vi "get_nxsp.vi"(5 "lc_num":string, 6 "yw":string, 7 "id":string, 9 "Cur_state":string, 11 "fqren":string) -> (1 "nx_state":dbl, 2 "sp_name":string, 3 "sp_gonghao":string)   [LabVIEW 2017, in "Lib_code.lvlib"]
uses:
  Lib_code.lvlib
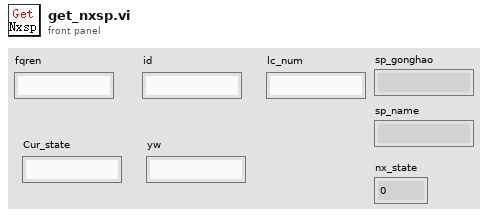
[diagram p1: front panel]
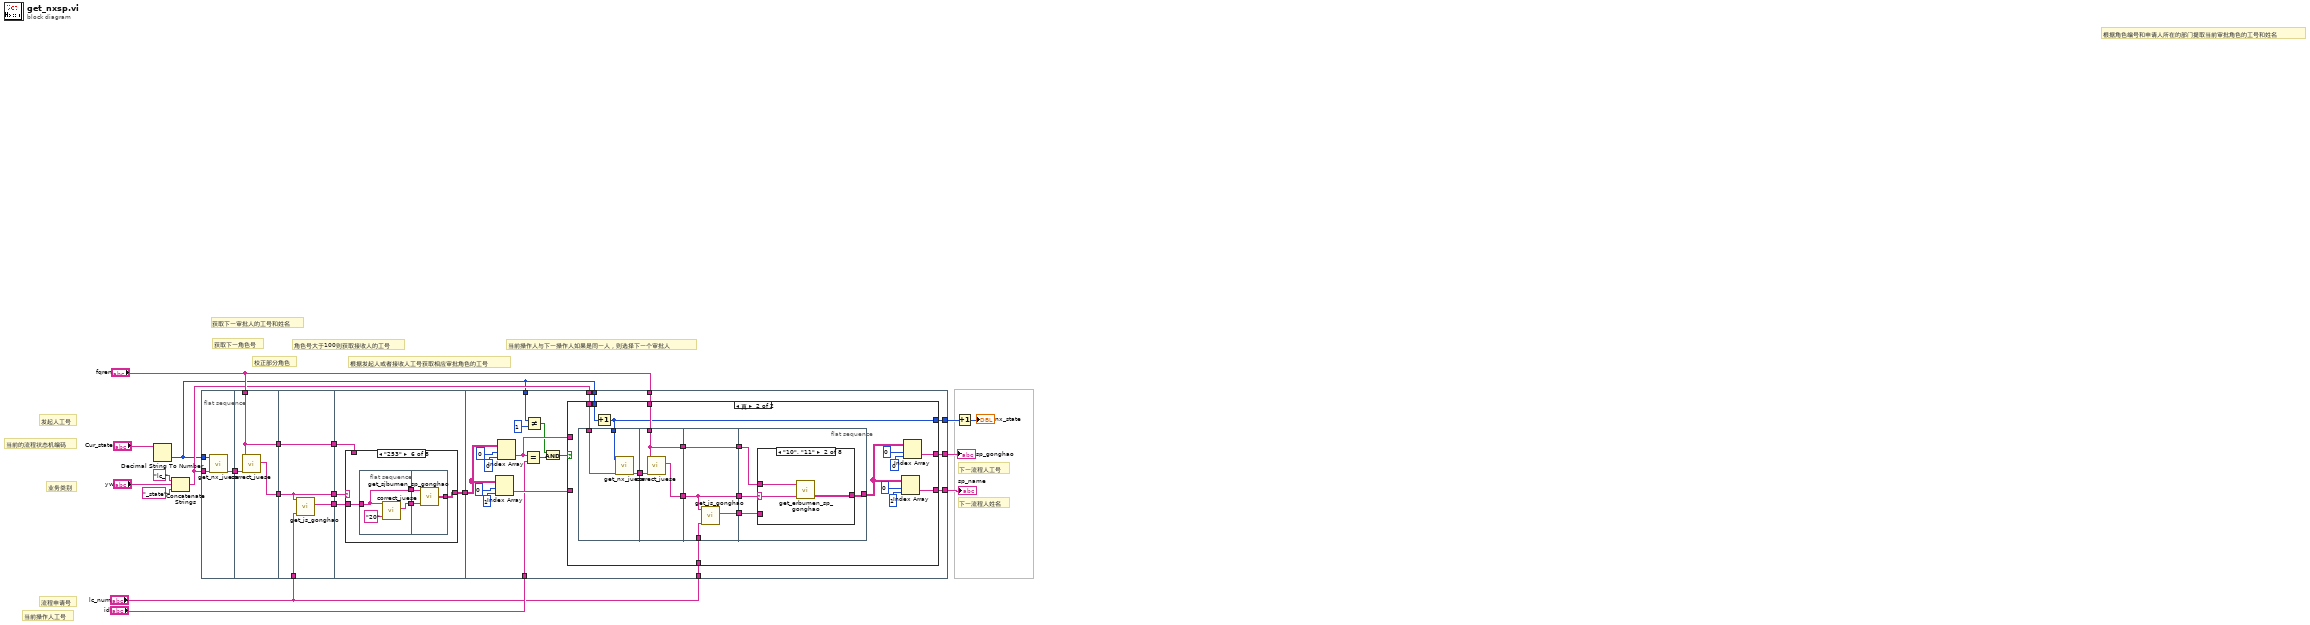
[diagram p0: block diagram]
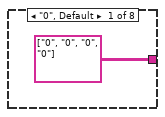
[diagram p2: hidden frame]
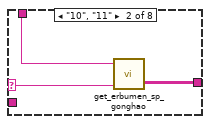
[diagram p3: hidden frame]
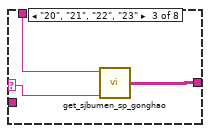
[diagram p4: hidden frame]
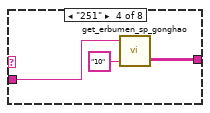
[diagram p5: hidden frame]
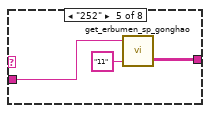
[diagram p6: hidden frame]
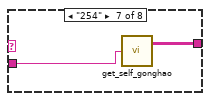
[diagram p7: hidden frame]
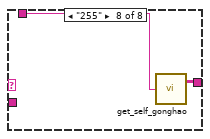
[diagram p8: hidden frame]
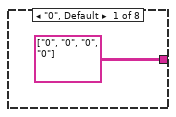
[diagram p10: hidden frame]
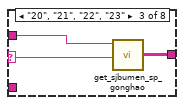
[diagram p11: hidden frame]
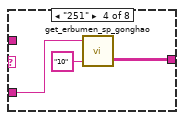
[diagram p12: hidden frame]
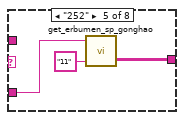
[diagram p13: hidden frame]
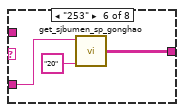
[diagram p14: hidden frame]
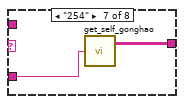
[diagram p15: hidden frame]
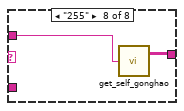
[diagram p16: hidden frame]
diagram:
  # "当前操作人与下一操作人如果是同一人，则选择下一个审批人"
  # "当前操作人工号"
  # "根据发起人或者接收人工号获取相应审批角色的工号"
  # "角色号大于100则获取接收人的工号"
  # "校正部分角色"
  # "获取下一角色号"
  # "流程申请号"
  # "发起人工号"
  # "下一流程人姓名"
  # "下一流程人工号"
  # "获取下一审批人的工号和姓名"
  # "业务类别"
  # "当前的流程状态机编码"
  # "根据角色编号和申请人所在的部门提取当前审批角色的工号和姓名"
  n1 = Decimal String To Number(string="Cur_state") -> (number=w1:i32)  [unwired: 2 in, 1 out]
  n2 = Concatenate Strings("lc_" ("字符串"), "yw", "_state" ("字符串")) -> (w7:string)
  n3 = flat-sequence {
    tunnel: w1 -> [w23]
    tunnel: w7 -> [w22]
    tunnel: [w21] -> w17
    tunnel: w17 -> [w26]
    tunnel: "fqren" -> [w24]
    tunnel: [w25] -> w16
    tunnel: [w24] -> w14
    tunnel: w16 -> [w28]
    tunnel: [w28] -> w15
    tunnel: w14 -> [w30]
    tunnel: [w30] -> w13
    tunnel: "lc_num" -> [w29]
    tunnel: [w27] -> w11
    tunnel: w15 -> [w34]
    tunnel: w13 -> [w33]
    tunnel: w11 -> [w31]
    tunnel: [w32] -> w10
    tunnel: w10 -> [w75]
    tunnel: "id" -> [w74]
    tunnel: "fqren" -> [w73]
    tunnel: w1 -> [w72]
    tunnel: w7 -> [w71]
    tunnel: "lc_num" -> [w70]
    tunnel: [w69] -> w5
    tunnel: [w68] -> w4
    tunnel: [w67] -> w2
    tunnel: w1 -> [w63]
    frame #0 {
      n4 = call "get_nx_juese.vi"("data_name"=w22, "state"=w23) -> ("nx_juese"=w21:string)  [unwired: 8 in, 1 out]
    }
    frame #1 {
      n5 = call "correct_juese.vi"("juese"=w26, "fqren"=w24) -> ("nx_juese"=w25:string)  [unwired: 6 in, 1 out]
    }
    frame #2 {
      n6 = call "get_js_gonghao.vi"("lc_num"=w29, "juese"=w28) -> ("jsren"=w27:string)  [unwired: 8 in, 1 out]
    }
    frame #3 {
      n7 = case shown="\"253\"" w34 {
        selector: w34 -> [_ w37 w40 _ _ _ _ _]
        tunnel: [string[][] [["0", "0"], ["0", "0"]] ("数组") w36 w41 w44 w47 w51 w59 w61] -> w32
        tunnel: w33 -> [_ w38 w39 _ _ _ _ w60]
        tunnel: w31 -> [_ _ _ w42 w46 w50 w58 _]
        frame "0", Default {
        }
        frame "10", "11" {
          n8 = call "get_erbumen_sp_gonghao.vi"("juese"=w37, "gonghao"=w38) -> ("sp"=w36:string[][])  [unwired: 1 in, 1 out]
        }
        frame "20", "21", "22", "23" {
          n9 = call "get_sjbumen_sp_gonghao.vi"("juese"=w40, "gonghao"=w39) -> ("sp"=w41:string[][])  [unwired: 3 in, 1 out]
        }
        frame "251" {
          n10 = call "get_erbumen_sp_gonghao.vi"("juese"="10", "gonghao"=w42) -> ("sp"=w44:string[][])  [unwired: 1 in, 1 out]
        }
        frame "252" {
          n11 = call "get_erbumen_sp_gonghao.vi"("juese"="11", "gonghao"=w46) -> ("sp"=w47:string[][])  [unwired: 1 in, 1 out]
        }
        frame "253" {
          n12 = flat-sequence {
            tunnel: w50 -> [w53]
            tunnel: [w53] -> w49
            tunnel: [w54] -> w48
            tunnel: [w57] -> w51
            tunnel: w49 -> [w56]
            tunnel: w48 -> [w55]
            frame #0 {
              n13 = call "correct_juese.vi"("juese"="20", "fqren"=w53) -> ("nx_juese"=w54:string)  [unwired: 6 in, 1 out]
            }
            frame #1 {
              n14 = call "get_sjbumen_sp_gonghao.vi"("juese"=w55, "gonghao"=w56) -> ("sp"=w57:string[][])  [unwired: 3 in, 1 out]
            }
          }
        }
        frame "254" {
          n15 = call "get_self_gonghao.vi"("gonghao"=w58) -> ("sp"=w59:string[][])  [unwired: 2 in, 1 out]
        }
        frame "255" {
          n16 = call "get_self_gonghao.vi"("gonghao"=w60) -> ("sp"=w61:string[][])  [unwired: 2 in, 1 out]
        }
      }
    }
    frame #4 {
      n17 = Index Array(array=w75, index (row)=0 ("索引 (行)"), index (col)=1 ("禁用的索引 (列)")) -> (element=w76:string)
      n18 = Index Array(array=w75, index (row)=0 ("索引 (行)"), index (col)=0 ("禁用的索引 (列)")) -> (element=w77:string)
      n19 = Equal?(x=w77, y=w74) -> (x = y?=w65:bool)
      n20 = Not Equal?(x=w63, y=1) -> (x != y?=w64:bool)
      n21 = And(x=w64, y=w65) -> (x .and. y?=w66:bool)
      n22 = case shown="真" w66 {
        tunnel: [w84 w88] -> w69
        tunnel: w77 -> [w84 _]
        tunnel: [w83 w90] -> w68
        tunnel: w76 -> [w83 _]
        tunnel: w72 -> [w82 w86]
        tunnel: w71 -> [_ w96]
        tunnel: w73 -> [_ w95]
        tunnel: w70 -> [_ w87]
        tunnel: [w82 w85] -> w67
        frame False {
        }
        frame True {
          n23 = flat-sequence {
            tunnel: [w105] -> w102
            tunnel: w96 -> [w104]
            tunnel: w85 -> [w103]
            tunnel: w102 -> [w108]
            tunnel: w95 -> [w106]
            tunnel: [w107] -> w101
            tunnel: [w106] -> w100
            tunnel: w101 -> [w110]
            tunnel: [w110] -> w99
            tunnel: w100 -> [w112]
            tunnel: [w112] -> w98
            tunnel: w87 -> [w111]
            tunnel: [w109] -> w97
            tunnel: w99 -> [w113]
            tunnel: w98 -> [w114]
            tunnel: [w116] -> w89
            tunnel: w97 -> [w115]
            frame #0 {
              n24 = call "get_nx_juese.vi"("data_name"=w104, "state"=w103) -> ("nx_juese"=w105:string)  [unwired: 8 in, 1 out]
            }
            frame #1 {
              n25 = call "correct_juese.vi"("juese"=w108, "fqren"=w106) -> ("nx_juese"=w107:string)  [unwired: 6 in, 1 out]
            }
            frame #2 {
              n26 = call "get_js_gonghao.vi"("lc_num"=w111, "juese"=w110) -> ("jsren"=w109:string)  [unwired: 8 in, 1 out]
            }
            frame #3 {
              n27 = case shown="\"10\", \"11\"" w113 {
                selector: w113 -> [_ w119 w121 _ _ _ _ _]
                tunnel: [string[][] [["0", "0"], ["0", "0"]] ("数组") w118 w122 w126 w129 w132 w134 w136] -> w116
                tunnel: w114 -> [_ w120 w123 _ _ _ _ w135]
                tunnel: w115 -> [_ _ _ w124 w128 w131 w133 _]
                frame "0", Default {
                }
                frame "10", "11" {
                  n28 = call "get_erbumen_sp_gonghao.vi"("juese"=w119, "gonghao"=w120) -> ("sp"=w118:string[][])  [unwired: 1 in, 1 out]
                }
                frame "20", "21", "22", "23" {
                  n29 = call "get_sjbumen_sp_gonghao.vi"("juese"=w121, "gonghao"=w123) -> ("sp"=w122:string[][])  [unwired: 3 in, 1 out]
                }
                frame "251" {
                  n30 = call "get_erbumen_sp_gonghao.vi"("juese"="10", "gonghao"=w124) -> ("sp"=w126:string[][])  [unwired: 1 in, 1 out]
                }
                frame "252" {
                  n31 = call "get_erbumen_sp_gonghao.vi"("juese"="11", "gonghao"=w128) -> ("sp"=w129:string[][])  [unwired: 1 in, 1 out]
                }
                frame "253" {
                  n32 = call "get_sjbumen_sp_gonghao.vi"("juese"="20", "gonghao"=w131) -> ("sp"=w132:string[][])  [unwired: 3 in, 1 out]
                }
                frame "254" {
                  n33 = call "get_self_gonghao.vi"("gonghao"=w133) -> ("sp"=w134:string[][])  [unwired: 2 in, 1 out]
                }
                frame "255" {
                  n34 = call "get_self_gonghao.vi"("gonghao"=w135) -> ("sp"=w136:string[][])  [unwired: 2 in, 1 out]
                }
              }
            }
          }
          n35 = Increment(x=w86) -> (x+1=w85:i32)
          n36 = Index Array(array=w89, index (row)=0 ("索引 (行)"), index (col)=1 ("禁用的索引 (列)")) -> (element=w90:string)
          n37 = Index Array(array=w89, index (row)=0 ("索引 (行)"), index (col)=0 ("禁用的索引 (列)")) -> (element=w88:string)
        }
      }
    }
  }
  n38 = Increment(x=w2) -> (x+1=→"nx_state":i32)
  "sp_gonghao" <- w5
  "sp_name" <- w4
